vi "SubVI_EXA get screen shot.vi"(8 "error in (no error)":errorcluster, 9 "File name":string, 10 "Path":path, 11 "VISA resource in":refnum<visa-resource-name>) -> (0 "error out":errorcluster, 3 "VISA resource out":refnum<visa-resource-name>)   [LabVIEW 2016]
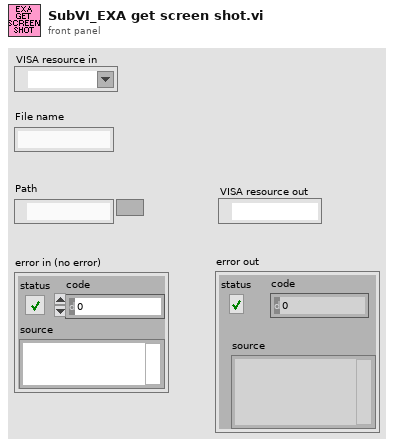
[diagram p1: front panel]
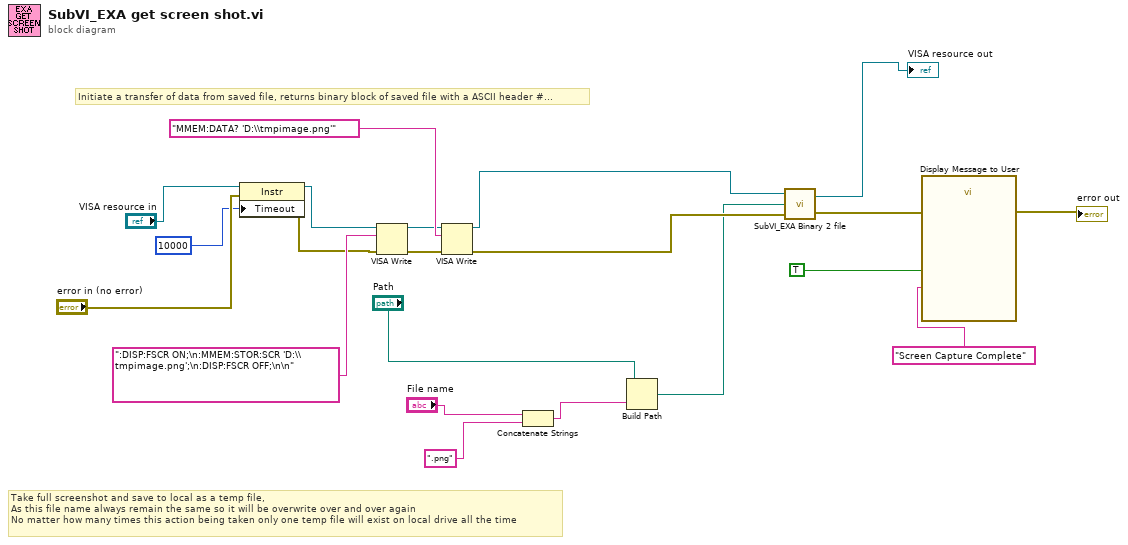
[diagram p0: block diagram]
diagram:
  # "Initiate a transfer of data from saved file, returns binary block of saved file with a ASCII header #..."
  # "Take full screenshot and save to local as a temp file, \nAs this file name always remain the same so it will be overwrite over and over again \nNo matter how many times this action being taken only one temp file will exist on local drive all the time"
  n1 = property class="Instr"(reference="VISA resource in", error in="error in (no error)", "Timeout"=u32 10000 ("General Settings:Timeout Value")) -> (reference out=w4:refnum<visa-resource-name>, error out=w2:errorcluster)
  n2 = VISA Write(VISA resource name=w4, write buffer=":DISP:FSCR ON;\n:MMEM:STOR:SCR 'D:\\tmpimage.png';\n:DISP:FSCR OFF;\n\n", error in (no error)=w2) -> (VISA resource name out=w15:refnum<visa-resource-name>, error out=w13:errorcluster)  [unwired: 1 out]
  n3 = VISA Write(VISA resource name=w15, write buffer="MMEM:DATA? 'D:\\tmpimage.png'", error in (no error)=w13) -> (VISA resource name out=w14:refnum<visa-resource-name>, error out=w7:errorcluster)  [unwired: 1 out]
  n4 = Concatenate Strings("File name", ".png") -> (w8:string)
  n5 = Build Path(base path="Path", name or relative path=w8) -> (appended path=w6:path)
  n6 = call "SubVI_EXA Binary 2 file.vi"("error in (no error)"=w7, "Path"=w6, "VISA resource in"=w14) -> ("error out"=w17:errorcluster, "VISA resource out"=→"VISA resource out":refnum<visa-resource-name>)
  n7 = call "Display Message to User"("error in (no error)"=w17, "Enable"=TRUE, "Message"="Screen Capture Complete") -> ("error out"=→"error out":errorcluster)  [unwired: 7 in, 1 out]
